vi "Siimulation - Make status.vi"(8 "error in (no error)":errorcluster, 11 "Status":T1) -> (0 "error out":errorcluster, 3 "Status":string)   [LabVIEW 2019, in "ACSVcontrol-driver.lvlib"]
doc: "For simulation: make a status message and sets it to status refnum, if available."
uses:
  ACSVcontrol-driver.lvlib
  Type definitions/Status.ctl
  Globals.vi
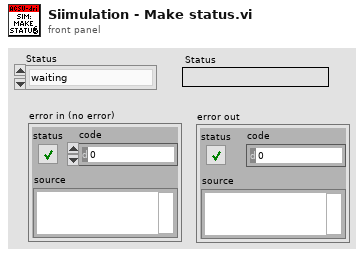
[diagram p1: front panel]
types:
  T1 = typedef "ACSVcontrol-driver.lvlib/Status.ctl" = enum16{"waiting", "processing", "error command", "Set_PJVS-Done", "Set_Mux-Done", "Set_Mux-Error", "Set_57XX-Done", "Set_57XX-Error", "Set_Gen-Done", "Set_Gen-Error", "Set_Synthesizer-Done", "Set_Synthesizer-Error", "Read_Nano-Done", "Read_Sampler-Done", "Read_Sampler-Error", "Read_Sensors-Done"}
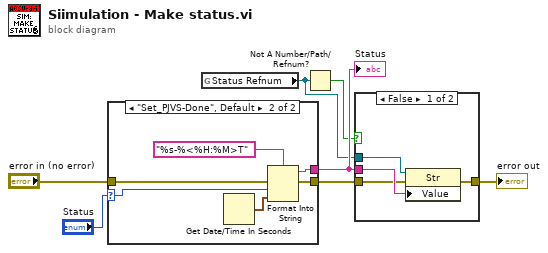
[diagram p0: block diagram]
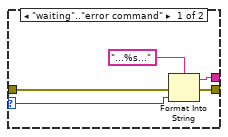
[diagram p2: hidden frame]
diagram:
  n1 = case shown="\"Set_PJVS-Done\", Default" "Status" {
    selector: "Status" -> [w11 w15]
    tunnel: [w10 w18] -> w7
    tunnel: "error in (no error)" -> [w9 w14]
    tunnel: [w8 w13] -> w2
    frame "waiting".."error command" {
      n2 = Format Into String(format string="...%s...", error in=w9, w11) -> (resulting string=w10:string, error out=w8:errorcluster)  [unwired: 1 in]
    }
    frame "Set_PJVS-Done", Default {
      n3 = Get Date/Time In Seconds() -> (seconds since 1Jan1904=w16:timestamp)
      n4 = Format Into String(format string="%s-%<%H:%M>T", error in=w14, w15, w16) -> (resulting string=w18:string, error out=w13:errorcluster)  [unwired: 1 in]
    }
  }
  "Status" <- w7
  n5 = global read "Globals.vi" "Status Refnum"() -> (w6:refnum<vi>)
  n6 = Not A Number/Path/Refnum?(number/path/refnum=w6) -> (NaN/Path/Refnum?=w5:bool)
  n7 = case shown="False" w5 {
    tunnel: w7 -> [w22 _]
    tunnel: w6 -> [w21 _]
    tunnel: w2 -> [w20 w23]
    tunnel: [w19 w23] -> w1
    frame False {
      n8 = property class="Str"(reference=w21, error in=w20, "Value"=w22) -> (error out=w19:errorcluster)  [unwired: 1 out]
    }
    frame True {
    }
  }
  "error out" <- w1
